vi "SENS_FOM_RANGE_SEGM_SWEEP_TIME_CONTROL.vi"(0 "VISA IN":refnum<visa-resource-name>, 1 "Range":i32, 2 "Enable Sweep Time? ON/OFF":bool, 5 "error in":errorcluster, 7 "Channel":i32) -> (14 "VISA Out":refnum<visa-resource-name>, 19 "error out":errorcluster)   [LabVIEW 2018, in "PNA-X.lvlib"]
uses:
  PNA-X.lvlib
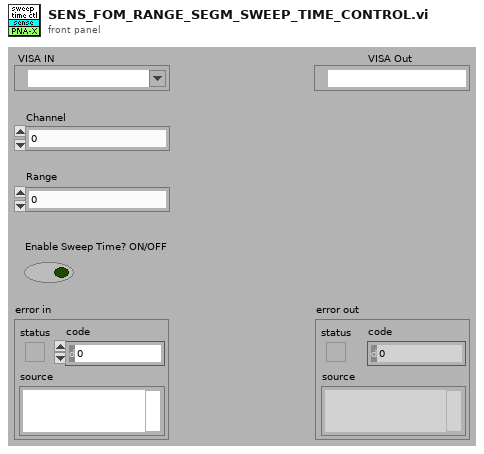
[diagram p1: front panel]
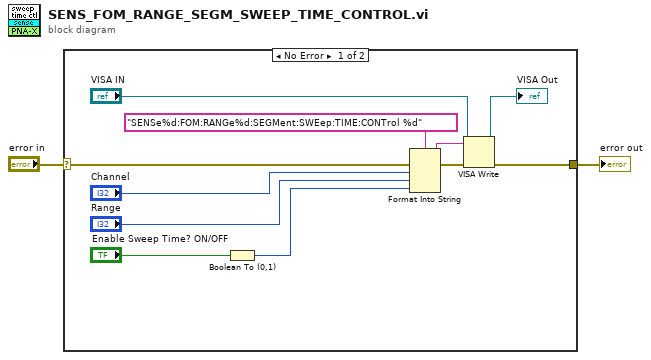
[diagram p0: block diagram]
diagram:
  n1 = case shown="No Error" "error in" {
    selector: "error in" -> [w13 w14]
    tunnel: [w8 w14] -> w1
    frame No Error {
      n2 = Boolean To (0,1)(Boolean="Enable Sweep Time? ON/OFF") -> (0, 1=w3:i16)
      n3 = Format Into String(format string="SENSe%d:FOM:RANGe%d:SEGMent:SWEep:TIME:CONTrol %d" ("Cmdline"), error in=w13, "Channel", "Range", w3) -> (resulting string=w11:string, error out=w12:errorcluster)  [unwired: 1 in]
      n4 = VISA Write(VISA resource name="VISA IN", write buffer=w11, error in (no error)=w12) -> (VISA resource name out=→"VISA Out":refnum<visa-resource-name>, error out=w8:errorcluster)  [unwired: 1 out]
    }
    frame Error {
    }
  }
  "error out" <- w1
